vi "Sort Conjugate Complex Numbers (Magnitude).vi"(10 "Order":enum16{"Ascending", "Descending"}(ring), 11 "Conjugate Complex Numbers":cdb[](array[numeric])) -> (3 "Sorted Conjugate Complex Numbers":cdb[](array[numeric]))   [LabVIEW 2020, in "NI_AALPro.lvlib"]
uses:
  NI_AALPro.lvlib
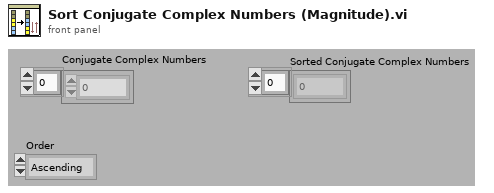
[diagram p1: front panel]
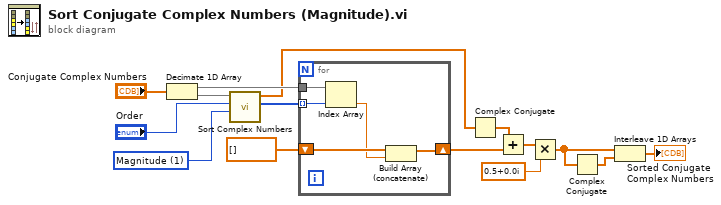
[diagram p0: block diagram]
diagram:
  w1 = u16 1 items=["Real & Imaginary", "Magnitude"] ("method")
  n1 = Decimate 1D Array("Conjugate Complex Numbers") -> (w11:cdb[], w13:cdb[])
  n2 = call "Sort Complex Numbers.vi"("method"=w1, "order"="Order", "Complex Numbers"=w13) -> ("Sorted Index"=w12:i32[], "Sorted Complex Numbers"=w8:cdb[])  [unwired: 6 in, 1 out]
  n3 = for {
    tunnel: w12 -> [w19] mode=indexing
    tunnel: w11 -> [w20]
    shift-right: [w16] -> w6
    shift-left: cdb[] [] -> [w18]
    n4 = Index Array(array=w20, index=w19) -> (element=w17:cdb)
    n5 = Build Array (concatenate)(w18, w17) -> (w16:cdb[])
  }
  n6 = Complex Conjugate(1:w8) -> (0:w7:cdb[])
  n7 = Add(x=w7, y=w6) -> (x+y=w5:cdb[])
  n8 = Multiply(x=w5, y=cdb 0.5+0.0i) -> (x*y=w3:cdb[])
  n9 = Complex Conjugate(1:w3) -> (0:w2:cdb[])
  n10 = Interleave 1D Arrays(w3, w2) -> (→"Sorted Conjugate Complex Numbers":cdb[])
